vi "NewPosCmd.vi"(8 "error in (no error)":errorcluster, 9 "AxisNumber":u8, 10 "NewPos-Data":T1, 11 "CS++Motor in":refnum<class "CS++Motor.lvclass">) -> (0 "error out":errorcluster, 3 "CS++Motor out":refnum<class "CS++Motor.lvclass">)   [LabVIEW 2015, in "CS++Motor.lvlib" / "CS++Motor.lvclass"]
uses:
  CS++Motor.lvclass
  CS++Motor.lvclass/CS++Motor.ctl
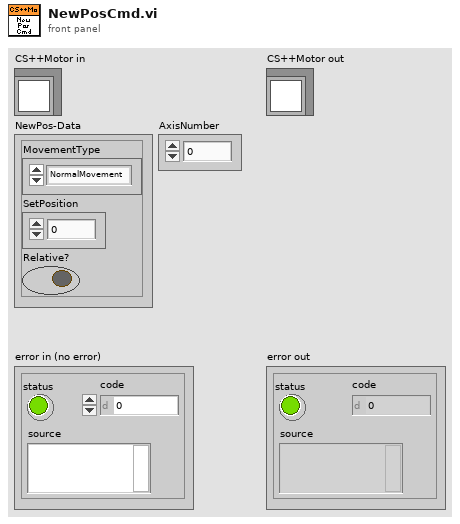
[diagram p1: front panel]
types:
  T1 = cluster{"MovementType":enum16{"NormalMovement", "ReferenceMovement", "StopMovement"}, "SetPosition":dbl, "Relative?":bool}
  T2 = cluster{"AxisNumber":u8, "RawSetPosition":dbl, "Relative?":bool, "RefMove?":bool}[]
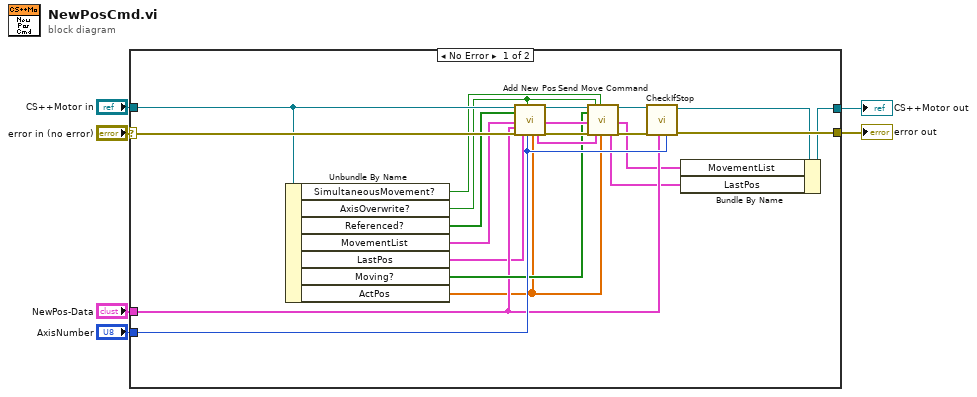
[diagram p0: block diagram]
diagram:
  n1 = case shown="No Error" "error in (no error)" {
    selector: "error in (no error)" -> [w22 w30]
    tunnel: [w21 w30] -> w5
    tunnel: [w11 w29] -> w3
    tunnel: "CS++Motor in" -> [w20 w29]
    tunnel: "AxisNumber" -> [w17 _]
    tunnel: "NewPos-Data" -> [w13 _]
    frame No Error {
      n2 = Unbundle By Name(w20) -> ("SimultaneousMovement?"=w15:bool, "AxisOverwrite?"=w16:bool, "Referenced?"=w18:bool[], "MovementList"=w19:T2, "LastPos"=w8:cluster{dbl[]}[], "Moving?"=w14:bool[], "ActPos"=w7:dbl[])
      n3 = call "Add New Pos.vi"("CS++Motor in"=w20, "Referenced"=w18, "MovementList In"=w19, "NewPos-Data"=w13, "error in (no error)"=w22, "LastPos In"=w8, "Axis Overwrite?"=w16, "AxisNumber"=w17, "ActPos"=w7) -> ("LastPos Out"=w23:cluster{dbl[]}[], "CS++Motor out"=w28:refnum<class "CS++Motor.lvclass">, "MovementList Out"=w26:T2, "error out"=w24:errorcluster)  [unwired: 7 in]
      n4 = call "Send Move Command.vi"("CS++Motor in"=w28, "Moving?"=w14, "MovementList In"=w26, "error in (no error)"=w24, "Axis Overwrite?"=w16, "LastPos In"=w23, "SimultaneousMovement?"=w15, "ActPos"=w7) -> ("LastPos Out"=w10:cluster{dbl[]}[], "CS++Motor out"=w27:refnum<class "CS++Motor.lvclass">, "MovementList Out"=w9:T2, "error out"=w25:errorcluster)  [unwired: 8 in]
      n5 = call "CheckIfStop.vi"("AxisNumber"=w17, "NewPos-Data"=w13, "error in (no error)"=w25, "CS++Motor in"=w27) -> ("error out"=w21:errorcluster, "CS++Motor out"=w12:refnum<class "CS++Motor.lvclass">)  [unwired: 6 in]
      n6 = Bundle By Name(cluster=w12, "MovementList"=w9, "LastPos"=w10) -> (w11:refnum<class "CS++Motor.lvclass">)
    }
    frame Error {
    }
  }
  "error out" <- w5
  "CS++Motor out" <- w3
